vi "GT Get Enc Response Check.vi"(0 "cardNum":i16, 1 "pTime":i32, 5 "control":i16, 7 "pDacThreshold":i16, 9 "pMinEncVel":dbl, 11 "error in (no error)":errorcluster caption="错误输入（无错误）") -> (3 "pTime out":i32, 4 "function return":i16, 8 "pDacThreshold out":i16, 10 "pMinEncVel out":dbl, 15 "error out":errorcluster caption="错误输出")   [LabVIEW 2014, in "gts.lvlib"]
doc: "GT_API GT_GetEncResponseCheck(short cardNum,short control,short *pDacThreshold,double *pMinEncVel,long *pTime);"
uses:
  gts.lvlib
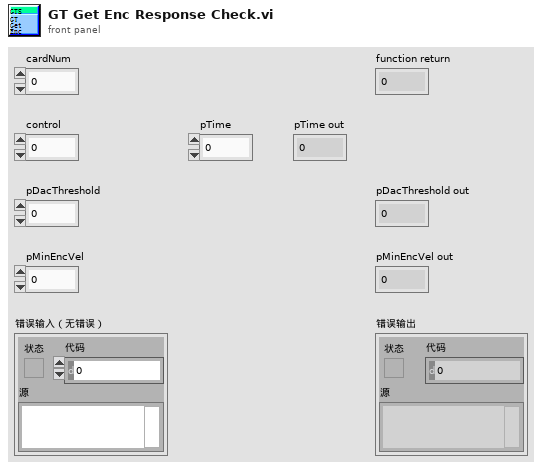
[diagram p1: front panel]
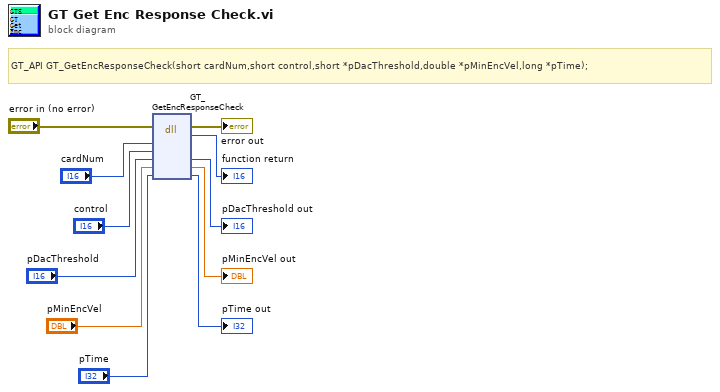
[diagram p0: block diagram]
diagram:
  # "GT_API GT_GetEncResponseCheck(short cardNum,short control,short *pDacThreshold,double *pMinEncVel,long *pTime);"
  n1 = dll-call lib="PTH2habs D固高科技资料GTS控制卡GTS卡18年上半年资料dllVC32bit\nmulti_cardgts.*" fn="GT_GetEncResponseCheck"(error in="error in (no error)", "cardNum"="cardNum", "control"="control", "pDacThreshold"="pDacThreshold", "pMinEncVel"="pMinEncVel", "pTime"="pTime") -> (error out=→"error out":errorcluster, →"function return":i16, "pDacThreshold"=→"pDacThreshold out":i16, "pMinEncVel"=→"pMinEncVel out":dbl, "pTime"=→"pTime out":i32)  [unwired: 4 in, 1 out]
